vi "Read Condition.vi"(11 "IL U16 Deny in":refnum<class "IL U16 Seize.lvclass">) -> (2 "Deny":u16[](array[numeric]), 3 "IL U16 Deny out":refnum<class "IL U16 Seize.lvclass">)   [LabVIEW 2015, in "Interlocks.lvlib" / "IL U16 Seize.lvclass"]
uses:
  IL U16 Seize.lvclass
  IL U16 Seize.lvclass/IL U16 Seize.ctl
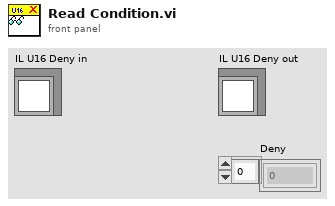
[diagram p1: front panel]
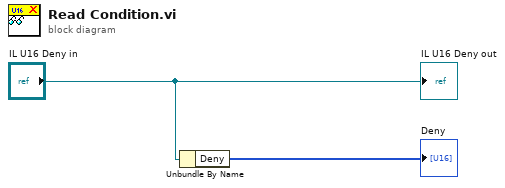
[diagram p0: block diagram]
diagram:
  n1 = Unbundle By Name("IL U16 Deny in") -> ("Deny"=→"Deny":u16[])
  "IL U16 Deny out" <- "IL U16 Deny in"
